vi "全局_配置.vi"() -> ()   [LabVIEW 2010]
panel:
  in  "R485路数":u32
  in  "ad模拟量输入路数":u32
  in  "dsp模拟量输入路数":u32
  out "CAN打开标志":bool
  in  "数字量输入路数":i32
  in  "数字量输出路数":i32
  in  "ARM模拟量量程范围":dbl
  in  "DSP模拟量量程范围":dbl
  in  "模拟量误差":dbl
  in  "超时时间_5":dbl
  in  "超时时间_10":dbl
  in  "超时时间_2":dbl
  in  "BoardConfig":T1
  in  "CAN端口":string(combo)
  in  "CAN波特率":u16
  in  "CAN发送帧数":u32
  in  "CAN数据":u8[](array[numeric]) format="%x"
  in  "RS232波特率":T2(ring)
  in  "R232路数":u32
  in  "本机IP":string
  in  "控制板端口":u16
  in  "本机端口":u16
  in  "控制板IP":string
  # "LAN设置"
  # "COM设置"
  # "CAN设置"
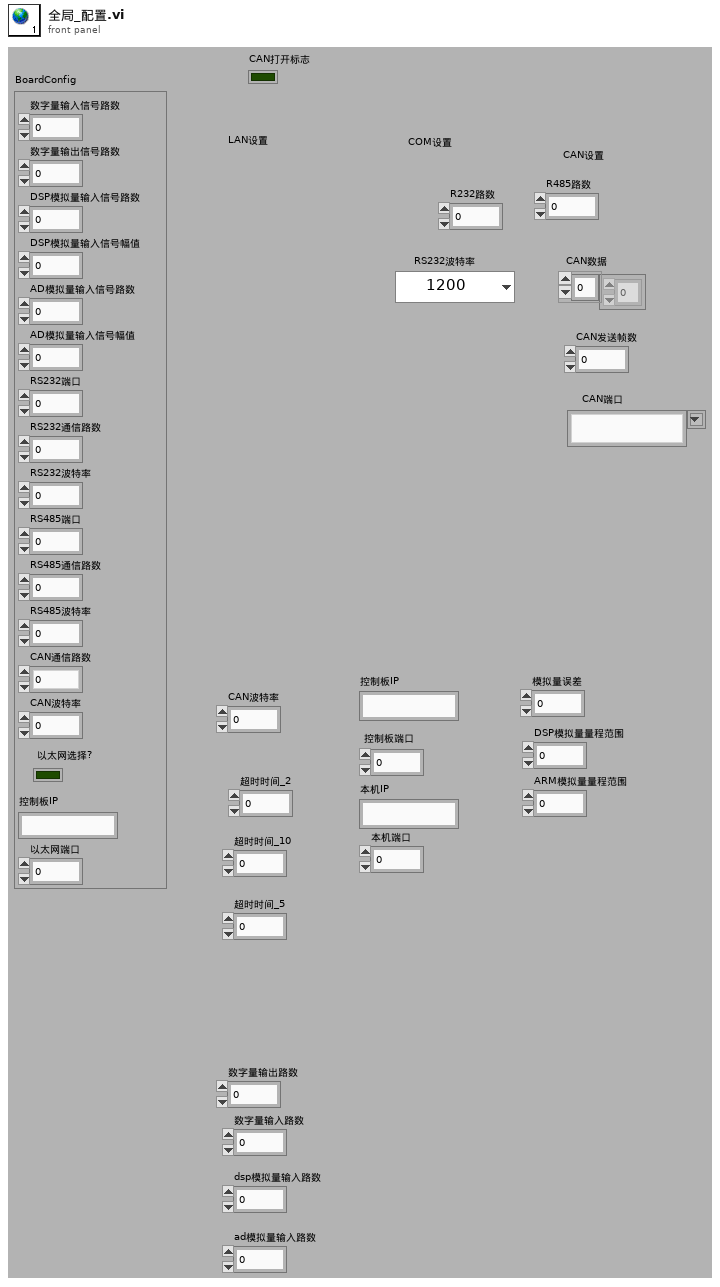
[diagram p1: front panel]
types:
  T1 = cluster{"数字量输入信号路数":u32, "数字量输出信号路数":u32, "DSP模拟量输入信号路数":u32, "DSP模拟量输入信号幅值":u32, "AD模拟量输入信号路数":u32, "AD模拟量输入信号幅值":u32, "RS232端口":i32, "RS232通信路数":u32, "RS232波特率":u32, "RS485端口":u32, "RS485通信路数":u32, "RS485波特率":u32, "CAN通信路数":i32, "CAN波特率":u32, "以太网选择?":bool, "控制板IP":string, "以太网端口":u32}
  T2 = enum32{"1200", "2400", "4800", "9600", "19200", "57600", "115200", ""}
diagram:
